vi "PassOrFail (SubVI).vi"(5 "Test#":string, 6 "String Res":string, 7 "index (row)":i32, 8 "error in (no error)":errorcluster, 9 "Data in":dbl format="%#_13g", 10 "Pass?Fail":bool, 11 "Table in":refnum<vi>) -> (0 "error out":errorcluster, 2 "Result":bool)   [LabVIEW 2017]
uses:
  <vilib>/Utility/miscctls.llb/LVRowAndColumnTypeDef.ctl
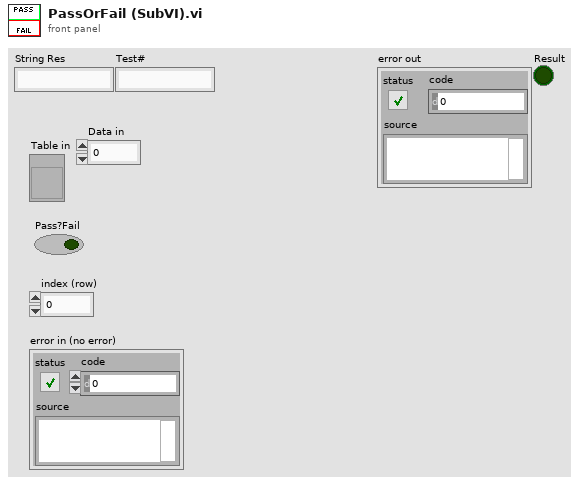
[diagram p1: front panel]
types:
  T1 = typedef "LVRowAndColumnTypeDef.ctl" = cluster{"Row":i32, "Column":i32}
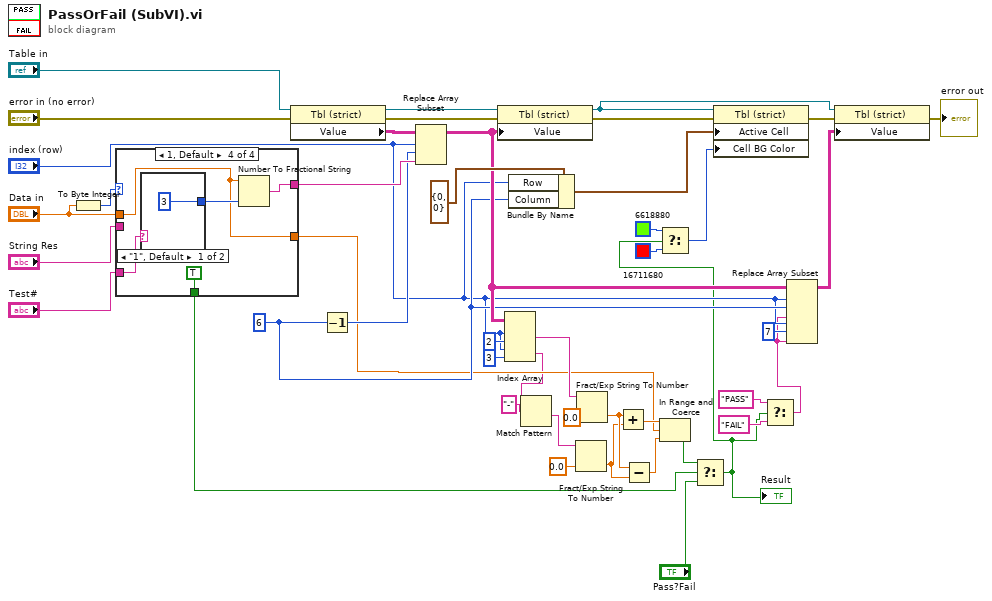
[diagram p0: block diagram]
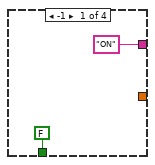
[diagram p2: hidden frame]
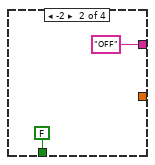
[diagram p3: hidden frame]
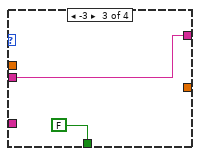
[diagram p4: hidden frame]
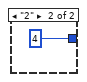
[diagram p5: hidden frame]
diagram:
  w20 = 6 ("disabled index (col)")
  n1 = To Byte Integer(number="Data in") -> (8bit integer=w26:i8)
  n2 = case shown="1, Default" w26 {
    tunnel: ["ON" "OFF" w51 w56] -> w29
    tunnel: "Data in" -> [_ _ _ w53]
    tunnel: "String Res" -> [_ _ w51 _]
    tunnel: "Test#" -> [_ _ _ w54]
    tunnel: [_ _ _ w53] -> w9
    tunnel: [FALSE FALSE FALSE TRUE] -> w4
    frame -1 {
    }
    frame -2 {
    }
    frame -3 {
    }
    frame 1, Default {
      n3 = case shown="\"1\", Default" w54 {
        tunnel: [i16 3 ("precision (6)") i16 4 ("precision (6)")] -> w55
        frame "1", Default {
        }
        frame "2" {
        }
      }
      n4 = Number To Fractional String(number=w53, precision (6)=w55) -> (F-format string=w56:string)  [unwired: 2 in]
    }
  }
  n5 = property class="Tbl (strict)"(reference="Table in", error in="error in (no error)") -> (reference out=w31:refnum<vi>, error out=w32:errorcluster, "Value"=w35:string[][])
  n6 = Decrement(x=w20) -> (x-1=w28:i32)
  n7 = Replace Array Subset(array=w35, new element=w29, index (row)="index (row)", index (col)=w28) -> (w21:string[][])
  n8 = property class="Tbl (strict)"(reference=w31, error in=w32, "Value"=w21) -> (reference out=w30:refnum<vi>, error out=w41:errorcluster)
  n9 = Index Array(array=w21, index (row) #1="index (row)", index (col) #1=2 ("disabled index (col)"), index (row) #2="index (row)", index (col) #2=3 ("disabled index (col)")) -> (element #1=w16:string, element #2=w7:string)
  n10 = Bundle By Name(cluster=T1 {"Row"=0, "Column"=0} ("Active Cell:Active Cell"), "Row"="index (row)", "Column"=w20) -> (w45:T1)
  n11 = Match Pattern(string=w7, regular expression="-") -> (after substring=w5:string)  [unwired: 1 in, 3 out]
  n12 = Fract/Exp String To Number(string=w5, default (0 dbl)=0.0 ("default (0 DBL)")) -> (number=w13:dbl)  [unwired: 2 in, 1 out]
  n13 = Fract/Exp String To Number(string=w16, default (0 dbl)=0.0 ("default (0 DBL)")) -> (number=w14:dbl)  [unwired: 2 in, 1 out]
  n14 = Add(x=w14, y=w13) -> (x+y=w15:dbl)
  n15 = Subtract(x=w14, y=w13) -> (x-y=w12:dbl)
  n16 = In Range and Coerce(upper limit=w15, x=w9, lower limit=w12) -> (In Range?=w2:bool)  [unwired: 1 out]
  n17 = Select(t=w2, s=w4, f="Pass?Fail") -> (s? t:f=w1:bool)
  "Result" <- w1
  n18 = Select(t=u32 6618880, s=w1, f=u32 16711680) -> (s? t:f=w39:u32)
  n19 = property class="Tbl (strict)"(reference=w30, error in=w41, "Active Cell"=w45, "Cell BG Color"=w39) -> (error out=w40:errorcluster)  [unwired: 1 out]
  n20 = Select(t="PASS" ("x"), s=w1, f="FAIL" ("x")) -> (s? t:f=w8:string)
  n21 = Replace Array Subset(array=w21, new element #1=w8, index (row) #1="index (row)", index (col) #1=w20, new element #2=w8, index (row) #2="index (row)", index (col) #2=7 ("disabled index (col)")) -> (w22:string[][])
  n22 = property class="Tbl (strict)"(reference=w30, error in=w40, "Value"=w22) -> (error out=→"error out":errorcluster)  [unwired: 1 out]
